vi "vclTimeToTimestamp.vi"(3 "all rows":dbl[](array[numeric])) -> (0 "before 2009?":bool, 1 "Array":timestamp[](array[timestamp]))   [LabVIEW 2019, in "VCL_2_DSC.lvclass"]
uses:
  VCL_2_DSC.lvclass
panel:
  out "x-y":dbl
  out "Numeric 2":dbl=2082844800.0 format="%#_10f"
  out "double precision float":dbl format="%#_10g"
  in  "time stamp 2":timestamp
  out "time stamp":timestamp
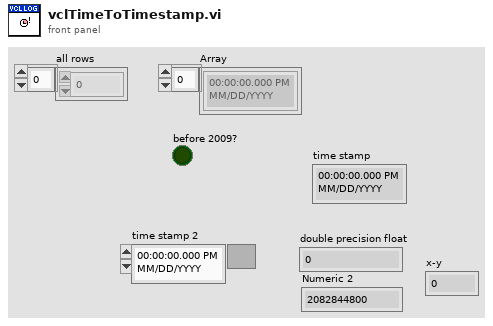
[diagram p1: front panel]
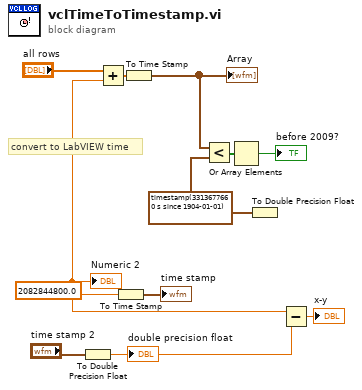
[diagram p0: block diagram]
diagram:
  w2 = 2082844800.0 ("Numeric 2")
  w1 = timestamp(3313677660 s since 1904-01-01)
  # "convert to LabVIEW time"
  n1 = To Double Precision Float(number="time stamp 2") -> (double precision float=w3:dbl)
  "double precision float" <- w3
  n2 = Add(x="all rows", y=w2) -> (x+y=w11:dbl[])
  n3 = To Time Stamp(1:w2) -> (0:→"time stamp":timestamp)
  n4 = To Time Stamp(1:w11) -> (0:w9:timestamp[])
  "Array" <- w9
  n5 = Less?(x=w9, y=w1) -> (x < y?=w8:bool[])
  n6 = Or Array Elements(Boolean array=w8) -> (logical OR=→"before 2009?":bool)
  n7 = To Double Precision Float(number=w1) -> ()  [unwired: 1 out]
  n8 = Subtract(x=w2, y=w3) -> (x-y=→"x-y":dbl)
  "Numeric 2" <- w2
